vi "move_stp.vi"(8 "error in (no error)":errorcluster caption="错误输入（无错误）", 10 "stp":i32, 11 "StepMotor 输入":refnum<class "StepMotor.lvclass">) -> (0 "error out":errorcluster caption="错误输出", 3 "StepMotor 输出":refnum<class "StepMotor.lvclass">)   [LabVIEW 2016, in "MotionControl_UFO_3DOF.lvlib" / "StepMotor.lvclass"]
uses:
  <userlib>/MotionControl_UFO_3DOF/StepMotor/StepMotor.lvclass
  <userlib>/MotionControl_UFO_3DOF/StepMotor/StepMotor.lvclass/StepMotor.ctl
  <userlib>/UISimCanFunc_wrapper/UISimCanFunc_wrapper.lvlib
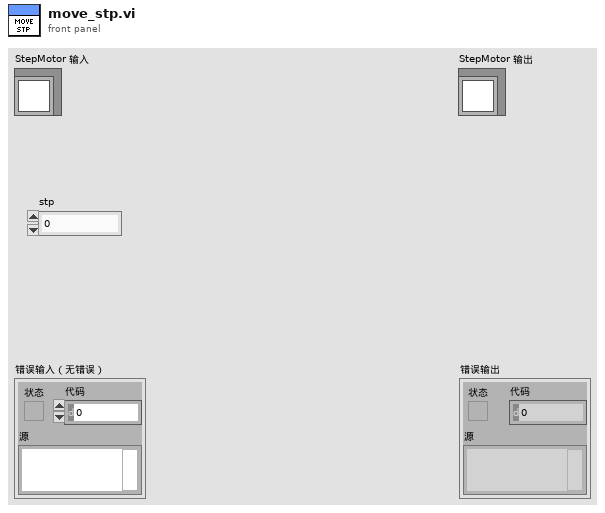
[diagram p1: front panel]
types:
  T1 = typedef "MotionControl_UFO_3DOF.lvlib/StepMotor.lvclass/AdvMovePara.ctl" = cluster{"acceleration":i32, "deceleration":i32, "max startup speed":i32, "max stop speed":i32}
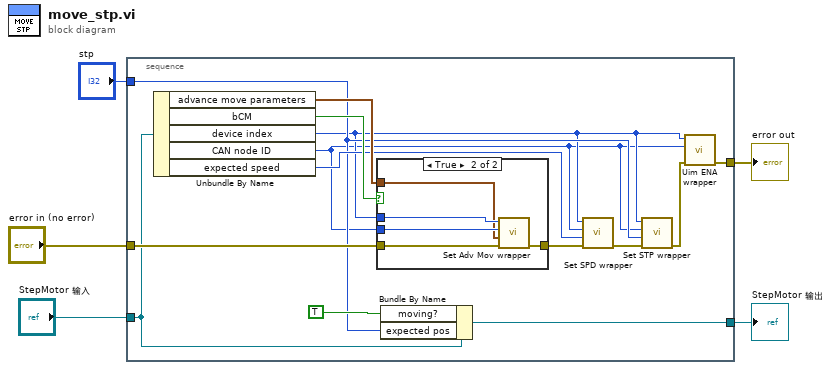
[diagram p0: block diagram]
diagram:
  n1 = stacked-sequence {
    tunnel: [w8] -> w2
    tunnel: [w18] -> w3
    tunnel: "StepMotor 输入" -> [w12]
    tunnel: "error in (no error)" -> [w17]
    tunnel: "stp" -> [w10]
    frame #0 {
      n2 = Unbundle By Name(w12) -> ("advance move parameters"=w16:T1, "bCM"=w19:bool, "device index"=w7:u32, "CAN node ID"=w6:u32, "expected speed"=w11:i32)
      n3 = case shown="True" w19 {
        tunnel: w7 -> [_ w25]
        tunnel: w6 -> [_ w24]
        tunnel: w17 -> [w20 w23]
        tunnel: [w20 w22] -> w15
        tunnel: w16 -> [_ w21]
        frame False {
        }
        frame True {
          n4 = call <userlib>:"Set Adv Mov wrapper.vi"("error in (no error)"=w23, "pAdvMovObj"=w21, "dwCanNodeId"=w24, "dwDevIndex"=w25) -> ("error out"=w22:errorcluster)  [unwired: 5 in, 2 out]
        }
      }
      n5 = Bundle By Name(cluster=w12, "moving?"=TRUE, "expected pos"=w10) -> (w18:refnum<class "StepMotor.lvclass">)
      n6 = call <userlib>:"Set SPD wrapper.vi"("error in (no error)"=w15, "iValue"=w11, "dwCanNodeId"=w6, "dwDevIndex"=w7) -> ("error out"=w14:errorcluster)  [unwired: 5 in, 2 out]
      n7 = call <userlib>:"Set STP wrapper.vi"("error in (no error)"=w14, "iValue"=w10, "dwCanNodeId"=w6, "dwDevIndex"=w7) -> ("error out"=w9:errorcluster)  [unwired: 5 in, 2 out]
      n8 = call <userlib>:"Uim ENA wrapper.vi"("error in (no error)"=w9, "dwCanNodeId"=w6, "dwDevIndex"=w7) -> ("error out"=w8:errorcluster)  [unwired: 6 in, 2 out]
    }
  }
  "error out" <- w2
  "StepMotor 输出" <- w3
